vi "Actor Core.vi"(8 "error in":errorcluster, 11 "Host Reply Time Test Actor in":refnum<class "Host Reply Time Test Actor.lvclass">) -> (0 "error out":errorcluster, 3 "Actor out":refnum<class "Actor.lvclass">)   [LabVIEW 2023, in "Host Reply Time Test Actor.lvlib" / "Host Reply Time Test Actor.lvclass"]
doc: "(<B>Filename</B>: Actor Framework.lvlib:Actor.lvclass:Actor Core.vi)\n\nReceives messages to the actor, reacts to them, and initiates any error handling that may shut the actor down.\n\nDescendant classes may override this VI to append parallel tasks for the actor to complete while it handles messages. Overrides use the Call Parent Class Method node."
uses:
  Host Reply Time Test Actor.lvclass
  C:/Program Files/National Instruments/LabVIEW 2023/vi.lib/ActorFramework/Actor/Actor.lvclass
  <vilib>/ActorFramework/Actor/Actor.lvclass
  <vilib>/ni/Actors/Network Endpoint Actors/Notifying Nested Endpoint/Notifying Nested Endpoint.lvclass
  C:/Program Files/National Instruments/LabVIEW 2023/vi.lib/ni/Actors/Network Endpoint Actors/Network Endpoint/Network Endpoint/Network Endpoint.lvclass
  Host Reply Time Test Actor.lvclass/Host Reply Time Test Actor.ctl
  <vilib>/ni/Actors/Network Endpoint Actors/Network Endpoint/Network Endpoint/Network Endpoint.lvclass/Network Endpoint.ctl
  <vilib>/ActorFramework/Actor/Actor.lvclass/Actor.ctl
  <vilib>/ActorFramework/Message Enqueuer/Message Enqueuer.lvclass/Message Enqueuer.ctl
  Target Reply Time Test Actor/Target Reply Time Test Actor Messages/Reply Msg DataSocket Msg/Reply Msg DataSocket Msg.lvclass/Reply Msg DataSocket Msg.ctl
  <vilib>/Analysis/baseanly.llb/Mean (DBL).vi
  <vilib>/ActorFramework/Message Enqueuer/Init from Existing Queue.vi
  <vilib>/ActorFramework/Message Enqueuer/Enqueue.vi
  Target Reply Time Test Actor/Target Reply Time Test Actor Messages/Reply Msg DataSocket Msg/Reply Msg DataSocket Msg.lvclass
  D:/git/Reply-Msg-DataSocket/Reply Msg DataSocket/Reply Msg DataSocket.lvclass
  Target Reply Time Test Actor/Target Reply Time Test Actor Messages/Shutdown Msg/Shutdown Msg.lvclass
  C:/Program Files/National Instruments/LabVIEW 2023/vi.lib/ActorFramework/Message/Message.lvclass
  <vilib>/ActorFramework/Stop Msg/Stop Msg.lvclass
  Reply Msg DataSocket/Send Message and Wait for Response.vi
  <vilib>/Utility/LVClass/Get LV Class Name.vi
  <resource>/AFDebug/Generate Trace for Message.vi
  <vilib>/ActorFramework/Message Priority Queue/Priority Enqueue.vi
  <vilib>/ActorFramework/Message Enqueuer/Message Enqueuer.lvclass
  <vilib>/ni/Actors/Network Endpoint Actors/Network Endpoint/Network Endpoint/Network Endpoint.lvclass
  <vilib>/Analysis/NI_AALBase.lvlib
  Reply Msg DataSocket/Reply Msg DataSocket.lvclass
panel:
  out "Waveform Chart":dbl(graph)
  out "mean":dbl format="%0.2f"
  out "error eventloop":errorcluster
  out "Response Times":dbl[](array[numeric])
  out "Replies":variant[](array[variant])
  out "Connected":bool
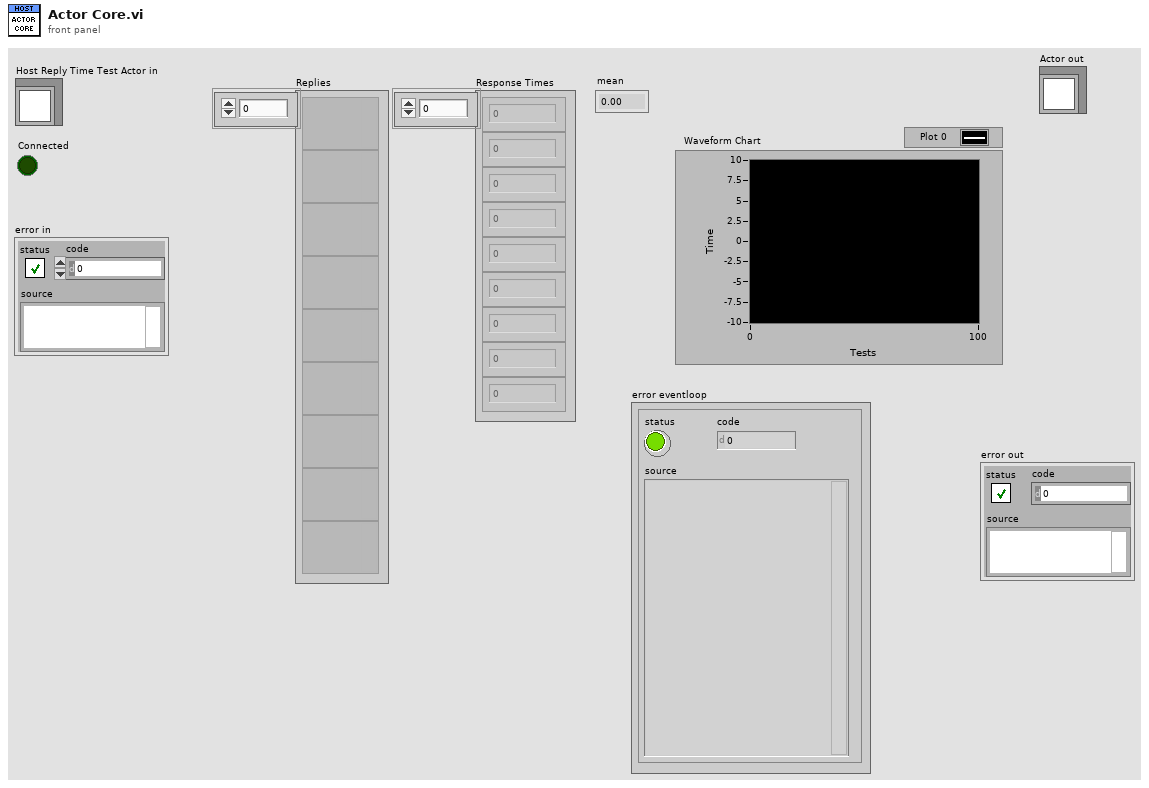
[diagram p1: front panel]
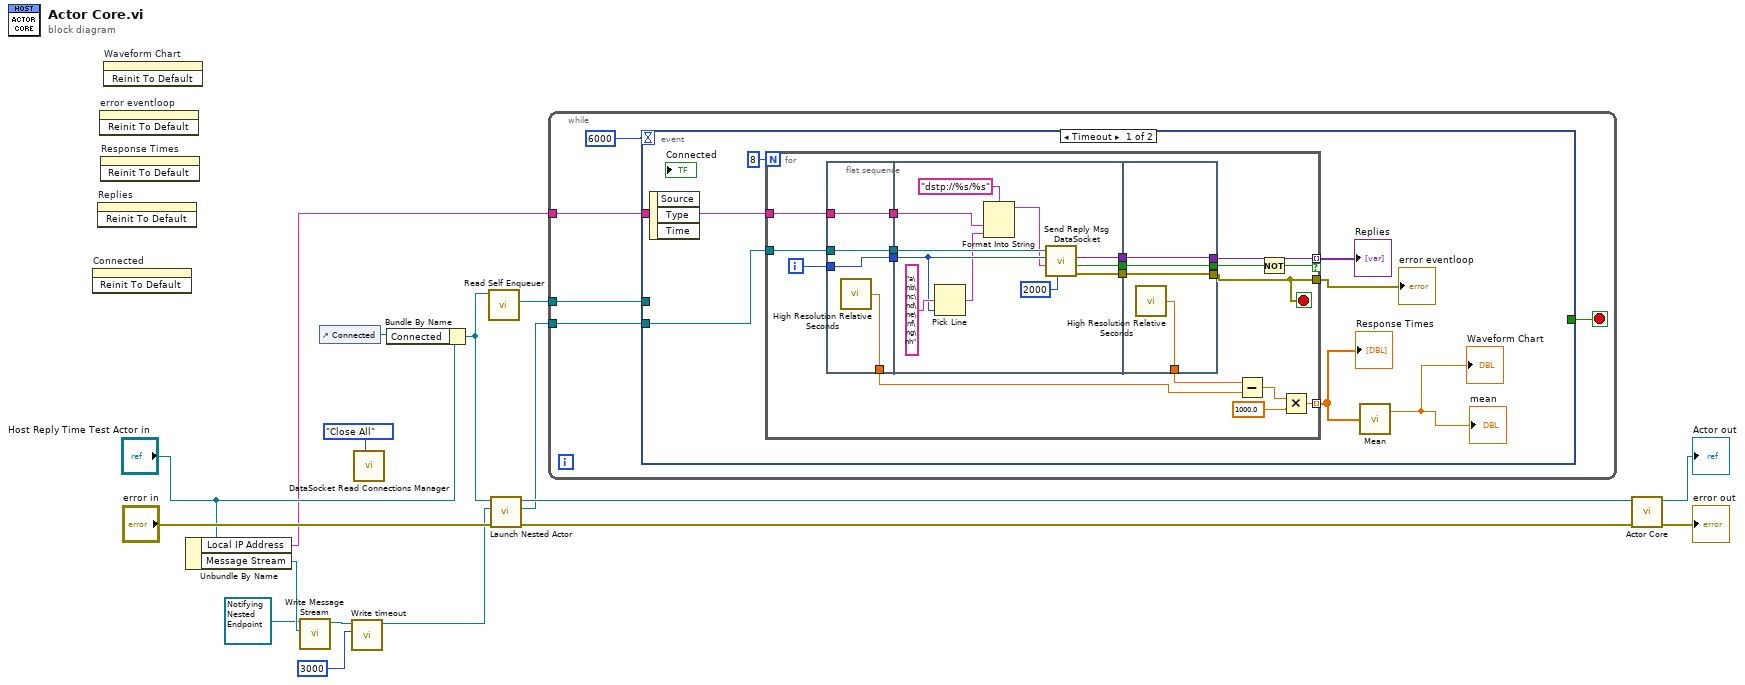
[diagram p0: block diagram]
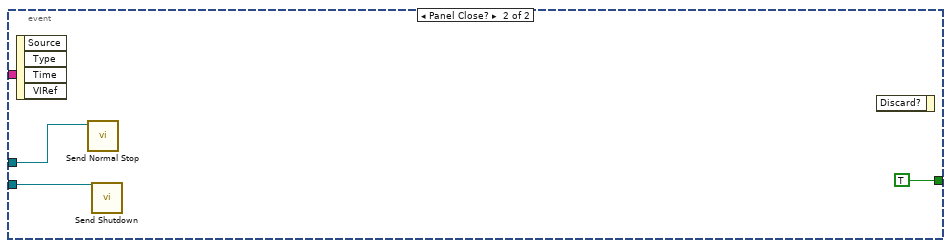
[diagram p2: hidden frame]
diagram:
  n1 = invoke on="Connected" class="Bool (strict)" method="Reinit To Default"() -> ()  [unwired: 3 in, 3 out]
  n2 = invoke on="Replies" class="Arr (strict)" method="Reinit To Default"() -> ()  [unwired: 3 in, 3 out]
  n3 = invoke on="error eventloop" class="Clust (strict)" method="Reinit To Default"() -> ()  [unwired: 3 in, 3 out]
  n4 = invoke on="Response Times" class="Arr (strict)" method="Reinit To Default"() -> ()  [unwired: 3 in, 3 out]
  n5 = invoke on="Waveform Chart" class="WFChart (strict)" method="Reinit To Default"() -> ()  [unwired: 3 in, 3 out]
  n6 = Unbundle By Name("Host Reply Time Test Actor in") -> ("Local IP Address"=w2:string, "Message Stream"=w11:refnum<class "Message Stream.lvclass">)
  n7 = call <vilib>:"Write Message Stream.vi"("Message Stream"=w11, "Network Endpoint in"=refnum<class "Notifying Nested Endpoint.lvclass"> refnum ("Notifying Nested Endpoint.lvclass")) -> ("Network Endpoint out"=w8:refnum<class "Notifying Nested Endpoint.lvclass">)  [unwired: 9 in]
  n8 = control-ref of="Connected"() -> (w13:refnum<vi>)
  n9 = call <vilib>:"Write timeout.vi"("timeout"=3000, "Network Endpoint in"=w8) -> ("Network Endpoint out"=w4:refnum<class "Notifying Nested Endpoint.lvclass">)  [unwired: 9 in]
  n10 = call "DataSocket Read Connections Manager.vi"("Action"=enum16{"Get", "Close", "Close All"}."Close All") -> ()  [unwired: 10 in, 1 out]
  n11 = Bundle By Name(cluster="Host Reply Time Test Actor in", "Connected"=w13) -> (w5:refnum<class "Host Reply Time Test Actor.lvclass">)
  n12 = call <vilib>:"Read Self Enqueuer.vi"("Actor"=w5) -> ("Self Enqueuer"=w14:refnum<class "Message Enqueuer.lvclass">)  [unwired: 10 in]
  n13 = call <vilib>:"Launch Nested Actor.vi"("error in (no error)"="error in", "Nested Actor"=w4, "Caller Actor in"=w5) -> ("error out"=w7:errorcluster, "Nested Actor's Enqueuer"=w3:refnum<class "Message Enqueuer.lvclass">, "Caller Actor out"=w6:refnum<class "Host Reply Time Test Actor.lvclass">)  [unwired: 6 in]
  n14 = while {
    tunnel: w14 -> [w22]
    tunnel: w3 -> [w20]
    tunnel: w2 -> [w18]
    stop <- w21 stop-if-true
    n15 = event shown="[0] Timeout" {
      selector: _ -> [_ _]
      dyn-events: _ -> [_ _]
      timeout: 6000 -> [_ _]
      tunnel: w22 -> [_ w69]
      tunnel: [_ TRUE] -> w21
      tunnel: w20 -> [w29 w67]
      tunnel: w18 -> [w24 _]
      event Timeout {
        n16 = event-data() -> ()  [unwired: 1 in, 3 out]
        n17 = for {
          N: 8 -> [_]
          tunnel: w29 -> [w47]
          tunnel: [w46] -> w28 mode=indexing if=w40
          tunnel: [w33] -> w25 mode=indexing
          tunnel: [w36] -> w26
          tunnel: w24 -> [w30]
          i -> [w39]
          stop <- w36 stop-if-true
          n18 = flat-sequence {
            tunnel: w47 -> [w51]
            tunnel: [w51] -> w44
            tunnel: [w50] -> w34
            tunnel: w39 -> [w49]
            tunnel: [w49] -> w38
            tunnel: [w48] -> w31
            tunnel: w30 -> [w48]
            tunnel: w44 -> [w62]
            tunnel: [w55] -> w43
            tunnel: [w54] -> w42
            tunnel: w38 -> [w57]
            tunnel: [w61] -> w37
            tunnel: w31 -> [w59]
            tunnel: [w65] -> w45
            tunnel: [w66] -> w46
            tunnel: w43 -> [w66]
            tunnel: w42 -> [w65]
            tunnel: [w64] -> w35
            tunnel: w37 -> [w63]
            tunnel: [w63] -> w36
            frame #0 {
              n19 = call <vilib>:"High Resolution Relative Seconds.vi"() -> ("relative seconds"=w50:dbl)
            }
            frame #1 {
              n20 = Pick Line(multi-line string="a\nb\nc\nd\ne\nf\ng\nh", line index=w57) -> (output string=w56:string)  [unwired: 1 in]
              n21 = Format Into String(format string="dstp://%s/%s", w59, w56) -> (resulting string=w52:string)  [unwired: 2 in, 1 out]
              n22 = call "Send Reply Msg DataSocket.vi"("Timeout"=2000, "DataSocket Reply URL"=w52, "Input"=w57, "Message Enqueuer"=w62) -> ("error out"=w61:errorcluster, "Timeout?"=w54:bool, "Reply"=w55:variant)  [unwired: 4 in, 1 out]
            }
            frame #2 {
              n23 = call <vilib>:"High Resolution Relative Seconds.vi"() -> ("relative seconds"=w64:dbl)
            }
          }
          n24 = Subtract(x=w35, y=w34) -> (x-y=w41:dbl)
          n25 = Not(x=w45) -> (.not. x?=w40:bool)
          n26 = Multiply(x=w41, y=1000.0) -> (x*y=w33:dbl)
        }
        "Replies" <- w28
        "Response Times" <- w25
        "error eventloop" <- w26
        n27 = call-poly <vilib>:"Mean.vi"("X"=w25) -> ("mean"=→"mean" →"Waveform Chart":dbl)  [unwired: 1 out]
      }
      event Panel Close? {
        n28 = event-data() -> ()  [unwired: 1 in, 4 out]
        n29 = call <vilib>:"Send Normal Stop.vi"("Message Enqueuer"=w69) -> ()  [unwired: 10 in, 1 out]
        n30 = call "Send Shutdown.vi"("Message Enqueuer"=w67) -> ()  [unwired: 9 in, 2 out]
        n31 = event-data() -> ()  [unwired: 2 in, 1 out]
      }
    }
  }
  n32 = call-parent "Actor Core.vi"("error in"=w7, "Actor in"=w6) -> ("error out"=→"error out":errorcluster, "Actor out"=→"Actor out":refnum<class "Actor.lvclass">)  [unwired: 8 in]
